vi "Get_Power.vi"(8 "error in (no error)":errorcluster, 11 "NKT in":refnum<class "NKT_Extreme.lvclass">) -> (0 "error out":errorcluster, 2 "Power":dbl, 3 "NKT out":refnum<class "NKT_Extreme.lvclass">)   [LabVIEW 2020, in "NKT_Extreme.lvclass"]
uses:
  <instrlib>/Classes/Laser/NKT/NKT_Extreme.lvclass
  <instrlib>/NKTP_API/NKTP_API.lvlib
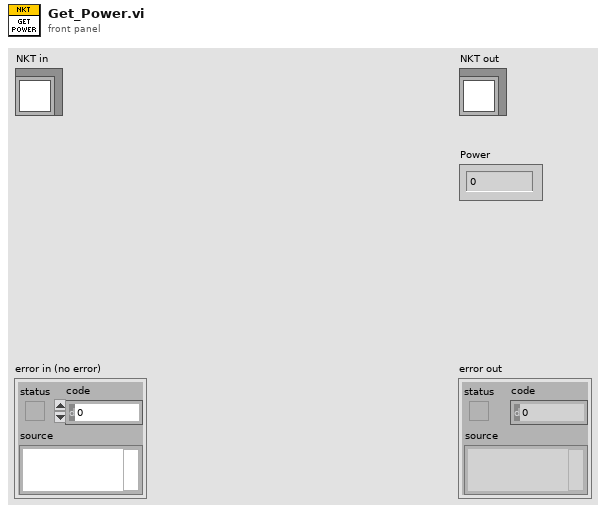
[diagram p1: front panel]
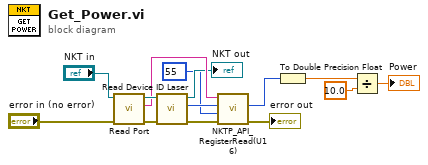
[diagram p0: block diagram]
diagram:
  n1 = call-dynamic "Read Port.vi"("error in (no error)"="error in (no error)", "NKT in"="NKT in") -> ("error out"=w12:errorcluster, "Port"=w10:string, "NKT out"=w13:refnum<class "NKT_Extreme.lvclass">)  [unwired: 7 in]
  n2 = call-dynamic "Read Device ID Laser.vi"("error in (no error)"=w12, "NKT in"=w13) -> ("error out"=w6:errorcluster, "Device ID Laser"=w9:u8, "NKT out"=→"NKT out":refnum<class "NKT_Extreme.lvclass">)  [unwired: 7 in]
  n3 = call <instrlib>:"NKTP_API_RegisterRead(U16).vi"("error in"=w6, "regId"=u8 55, "devId"=w9, "portname"=w10) -> ("error out"=→"error out":errorcluster, "value"=w4:u16)  [unwired: 5 in, 1 out]
  n4 = To Double Precision Float(number=w4) -> (double precision float=w2:dbl)
  n5 = Divide(x=w2, y=10.0) -> (x/y=→"Power":dbl)
